vi "Scale Preview Picture.vi"(8 "error in (no error)":errorcluster, 10 "Accessors:Preview2":T1, 11 "Picture in":refnum<vi>) -> (0 "error out":errorcluster)   [LabVIEW 2015, in "Item Actor.lvlib" / "Instrument.lvclass"]
uses:
  Instrument.lvclass
  <vilib>/picture/picture.llb/imagedata.ctl
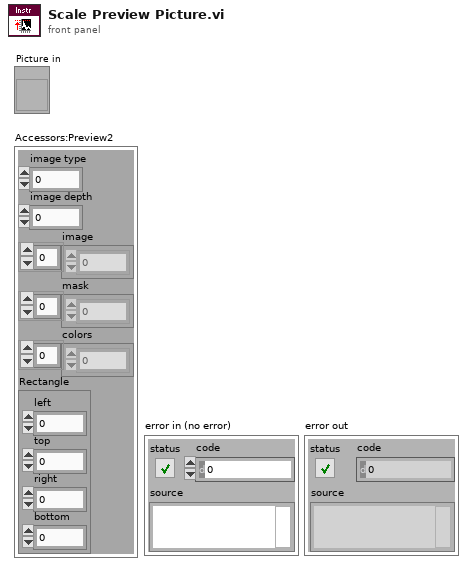
[diagram p1: front panel]
types:
  T1 = typedef "imagedata.ctl" = cluster{"image type":i32, "image depth":i32, "image":u8[], "mask":u8[], "colors":u32[], "Rectangle":cluster{"left":i16, "top":i16, "right":i16, "bottom":i16}}
  T2 = typedef "LVBoundsTypeDef.ctl" = cluster{"Width":u32, "Height":u32}
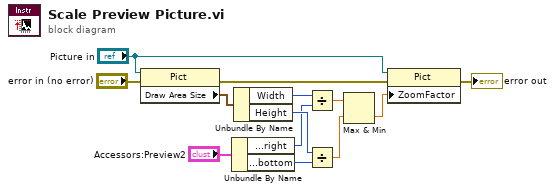
[diagram p0: block diagram]
diagram:
  n1 = property on="Property Node" class="Pict"(reference="Picture in", error in="error in (no error)") -> (error out=w2:errorcluster, "Draw Area Size"=w6:T2)  [unwired: 1 out]
  n2 = Unbundle By Name("Accessors:Preview2") -> ("Rectangle.right"=w7:i16, "Rectangle.bottom"=w9:i16)
  n3 = Unbundle By Name(w6) -> ("Width"=w8:u32, "Height"=w10:u32)
  n4 = Divide(x=w8, y=w7) -> (x/y=w12:dbl)
  n5 = Divide(x=w10, y=w9) -> (x/y=w11:dbl)
  n6 = Max & Min(x=w12, y=w11) -> (min(x,y)=w13:dbl)  [unwired: 1 out]
  n7 = property on="Property Node" class="Pict"(reference="Picture in", error in=w2, "ZoomFactor"=w13) -> (error out=→"error out":errorcluster)  [unwired: 1 out]
